vi "MaxMinDecimate.vi"(10 "decimation factor":i32, 11 "Array":sgl[](array[numeric]) format="%.2f") -> (1 "actual decimation":sgl format="%.2f", 2 "decimated array":sgl[](array[numeric]) format="%.2f", 3 "dup Array":sgl[](array[numeric]) format="%.2f")   [LabVIEW 2019]
doc: "Decimate an array before it is sent to the graph object so that processing time and memory are saved."
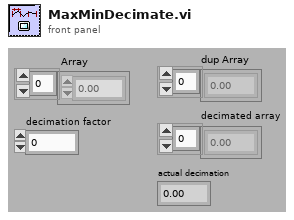
[diagram p1: front panel]
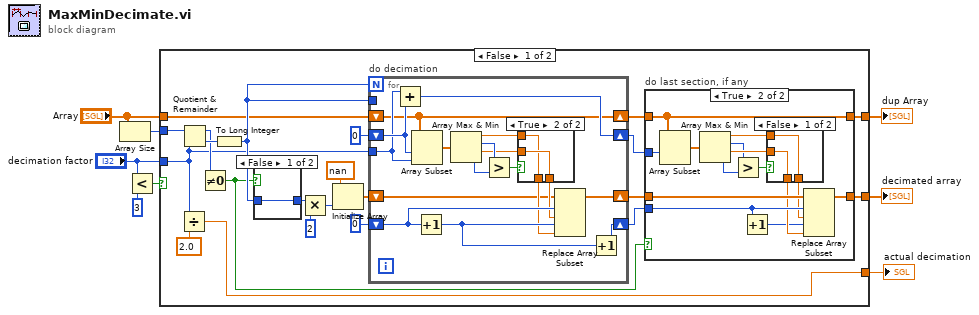
[diagram p0: block diagram]
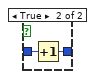
[diagram p4: hidden frame]
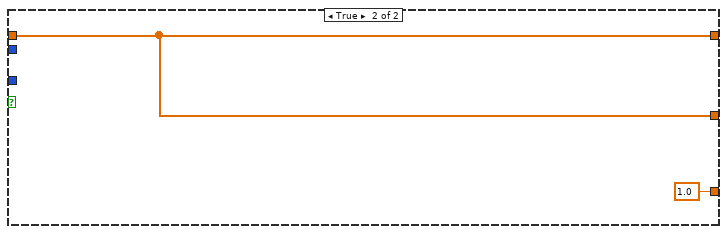
[diagram p6: hidden frame]
diagram:
  n1 = Array Size(array="Array") -> (size(s)=w3:i32)
  n2 = Less?(x="decimation factor", y=3) -> (x < y?=w7:bool)
  n3 = case shown="False" w7 {
    tunnel: "Array" -> [w10 w75]
    tunnel: [w15 w75] -> w5
    tunnel: [w21 w75] -> w4
    tunnel: "decimation factor" -> [w13 _]
    tunnel: w3 -> [w28 _]
    tunnel: [w11 sgl 1.0 ("actual decimation")] -> w1
    frame False {
      n4 = Divide(x=w13, y=sgl 2.0) -> (x/y=w11:sgl)
      n5 = Quotient & Remainder(x=w28, y=w13) -> (x-y*floor(x/y)=w18:i32, floor(x/y)=w19:i32)
      n6 = Not Equal To 0?(x=w18) -> (x != 0?=w14:bool)
      n7 = To Long Integer(number=w19) -> (32bit integer=w16:i32)
      n8 = case shown="False" w14 {
        tunnel: [w51 w53] -> w17
        tunnel: w16 -> [w51 w52]
        frame False {
        }
        frame True {
          n9 = Increment(x=w52) -> (x+1=w53:i32)
        }
      }
      n10 = Multiply(x=w17, y=2) -> (x*y=w25:i32)
      n11 = Initialize Array(sgl nan, w25) -> (w24:sgl[])
      n12 = for "do decimation" {
        N: w16 -> [_]
        shift-right: [w69] -> w20
        shift-left: 0 ("32bit integer") -> [w70]
        shift-right: [w55] -> w23
        shift-left: 0 ("32bit integer") -> [w66]
        tunnel: w16 -> [_]
        tunnel: w13 -> [w58]
        shift-right: [w56] -> w22
        shift-left: w24 -> [w57]
        shift-right: [w54] -> w9
        shift-left: w10 -> [w54]
        n13 = Add(x=w58, y=w66) -> (x+y=w55:i32)
        n14 = Array Subset(array=w54, index=w66, length=w58) -> (w67:sgl[])
        n15 = Increment(x=w70) -> (x+1=w68:i32)
        n16 = Array Max & Min(array=w67) -> (max value=w61:sgl, max index (indices)=w64:i32, min value=w62:sgl, min index (indices)=w63:i32)
        n17 = Greater?(x=w64, y=w63) -> (0:w65:bool)
        n18 = case shown="True" w65 {
          tunnel: w62 -> [w71 w74]
          tunnel: w61 -> [w72 w73]
          tunnel: [w72 w74] -> w60
          tunnel: [w71 w73] -> w59
          frame False {
          }
          frame True {
          }
        }
        n19 = Replace Array Subset(array=w57, new element #1=w60, index #1=w70, new element #2=w59, index #2=w68) -> (w56:sgl[])
        n20 = Increment(x=w68) -> (x+1=w69:i32)
      }
      n21 = case "do last section, if any" shown="True" w14 {
        tunnel: w23 -> [_ w46]
        tunnel: w9 -> [w32 w34]
        tunnel: w22 -> [w31 w45]
        tunnel: [w31 w33] -> w21
        tunnel: w20 -> [_ w43]
        tunnel: [w32 w34] -> w15
        frame False {
        }
        frame True {
          n22 = Array Subset(array=w34, index=w46) -> (w44:sgl[])  [unwired: 1 in]
          n23 = Array Max & Min(array=w44) -> (max value=w41:sgl, max index (indices)=w38:i32, min value=w40:sgl, min index (indices)=w39:i32)
          n24 = Greater?(x=w38, y=w39) -> (0:w37:bool)
          n25 = Increment(x=w43) -> (x+1=w35:i32)
          n26 = case shown="False" w37 {
            tunnel: w40 -> [w47 w50]
            tunnel: w41 -> [w48 w49]
            tunnel: [w48 w50] -> w42
            tunnel: [w47 w49] -> w36
            frame False {
            }
            frame True {
            }
          }
          n27 = Replace Array Subset(array=w45, new element #1=w42, index #1=w43, new element #2=w36, index #2=w35) -> (w33:sgl[])
        }
      }
    }
    frame True {
    }
  }
  "dup Array" <- w5
  "decimated array" <- w4
  "actual decimation" <- w1
